vi "GD_GWID5F_info.vi"(8 "error in (no error)":errorcluster, 9 "evaluation_1":i16=1, 10 "glue_id":string, 11 "DBlink":string="Driver={ODBC Driver 17 for SQL Server};Server=localhost\\SQLEXPRESS;Database=ZDX201;UID=labview;PWD=Dsa@54137926") -> (0 "error out":errorcluster)   [LabVIEW 2019]
uses:
  <vilib>/addons/database/Auxilliary.llb/DB Tools Format Datetime String (Time Stamp).vi
  <vilib>/addons/database/Connection.llb/DB Tools Open Connec (String).vi
  <vilib>/addons/database/NI_Database_API.lvlib
panel:
  out "Boolean array":bool[](array[boolean])
  out "Result":string
  out "Command 2":string="WHERE [id]=16"
  in  "columns":string[](array[string])=["evaluation_1", "update_time", "eve_finish_1"]
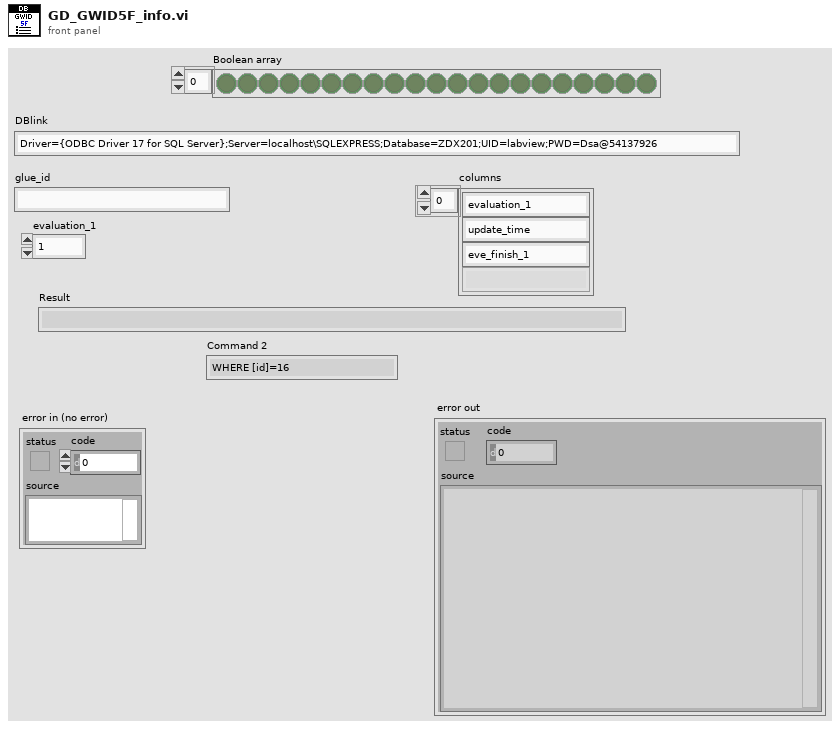
[diagram p1: front panel]
types:
  T1 = cluster{"evaluation_1":string, "update_time":timestamp, "eve_finish_1":timestamp}
  T2 = typedef "NI_Database_API.lvlib/Conn ObjectReference.ctl" = refnum<k1>
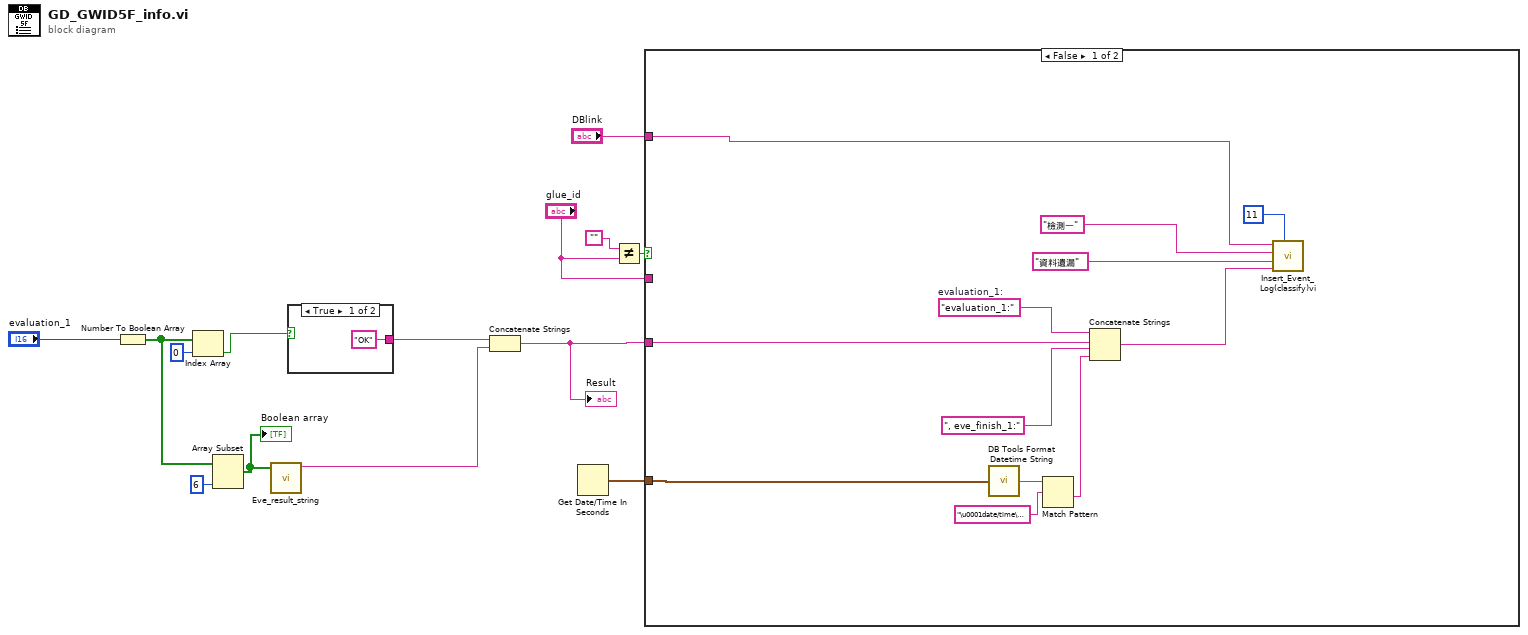
[diagram p0: block diagram]
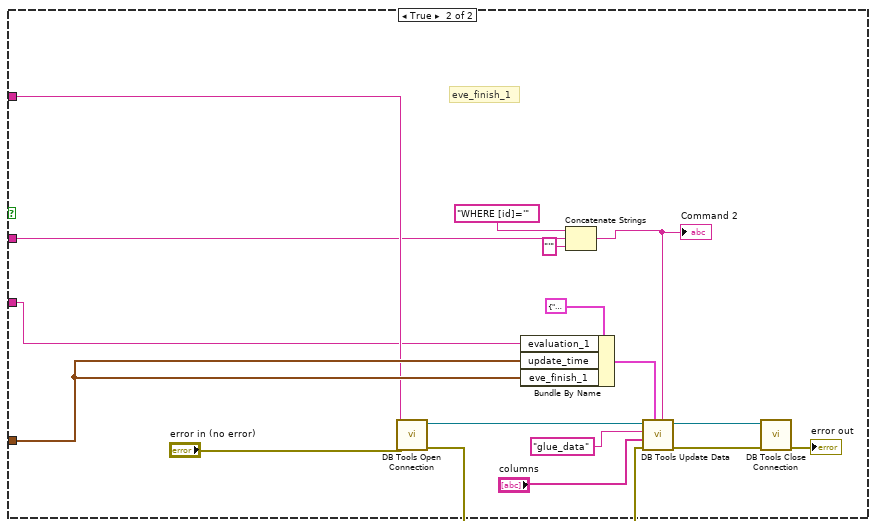
[diagram p2: hidden frame]
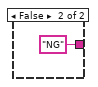
[diagram p3: hidden frame]
diagram:
  n1 = Number To Boolean Array(number="evaluation_1") -> (Boolean array=w3:bool[])
  n2 = Index Array(array=w3, index=0) -> (element=w7:bool)
  n3 = Array Subset(array=w3, length=6) -> (w2:bool[])  [unwired: 1 in]
  "Boolean array" <- w2
  n4 = call "Eve_result_string.vi"("Boolean array"=w2) -> ("String"=w1:string)  [unwired: 10 in]
  n5 = case shown="True" w7 {
    tunnel: ["OK" "NG"] -> w6
    frame True {
    }
    frame False {
    }
  }
  n6 = Concatenate Strings(w6, w1) -> (w5:string)
  "Result" <- w5
  n7 = Get Date/Time In Seconds() -> (seconds since 1Jan1904=w14:timestamp)
  n8 = Not Equal?(x="", y="glue_id") -> (x != y?=w10:bool)
  n9 = case shown="False" w10 {
    tunnel: w14 -> [w19 w36]
    tunnel: "DBlink" -> [w20 w32]
    tunnel: "glue_id" -> [_ w30]
    tunnel: w5 -> [w17 w29]
    frame False {
      w18 = "evaluation_1:"  # evaluation_1:
      n10 = call-poly <vilib>:"DB Tools Format Datetime String.vi"("time stamp"=w19) -> ("date/time string"=w25:string)
      n11 = Match Pattern(string=w25, regular expression="\u0001date/time\u0001" ("search string")) -> (after substring=w23:string)  [unwired: 1 in, 3 out]
      n12 = Concatenate Strings(w18, w17, ", eve_finish_1:", w23) -> (w22:string)
      n13 = call "Insert_Event_Log(classify)vi.vi"("classify"=i16 11, "data"=w22, "message"="資料遺漏", "id"="檢測一", "DBlink"=w20) -> ()  [unwired: 6 in, 1 out]
    }
    frame True {
      # "eve_finish_1"
      n14 = call-poly <vilib>:"DB Tools Open Connection.vi"("error in (no error)"="error in (no error)", "connection information"=w32) -> ("error out"=w44:errorcluster, "connection reference"=w37:T2)  [unwired: 6 in]
      n15 = Bundle By Name(cluster=T1 {"evaluation_1"="", "update_time"=timestamp(0 s since 1904-01-01), "eve_finish_1"=timestamp(0 s since 1904-01-01)}, "evaluation_1"=w29, "update_time"=w36, "eve_finish_1"=w36) -> (w38:T1)
      n16 = Concatenate Strings("WHERE [id]='", w30, "'" ("string")) -> (w33:string)
      "Command 2" <- w33
      n17 = call <vilib>:"DB Tools Update Data.vi"("condition"=w33, "data"=w38, "error in (no error)"=w44, "columns"="columns", "table"="glue_data", "connection reference"=w37) -> ("error out"=w45:errorcluster, "connection reference out"=w43:T2)  [unwired: 4 in]
      n18 = call <vilib>:"DB Tools Close Connection.vi"("error in (no error)"=w45, "connection reference"=w43) -> ("error out"=→"error out":errorcluster)  [unwired: 5 in]
    }
  }
